vi "TEST.vi"() -> ()   [LabVIEW 2017]
uses:
  <vilib>/Utility/miscctls.llb/LVPointTypeDef.ctl
  <vilib>/Utility/miscctls.llb/LVBoundsTypeDef.ctl
  <vilib>/Utility/miscctls.llb/LVRectTypeDef.ctl
panel:
  in  "stop":bool
  out "PictureBox":picture
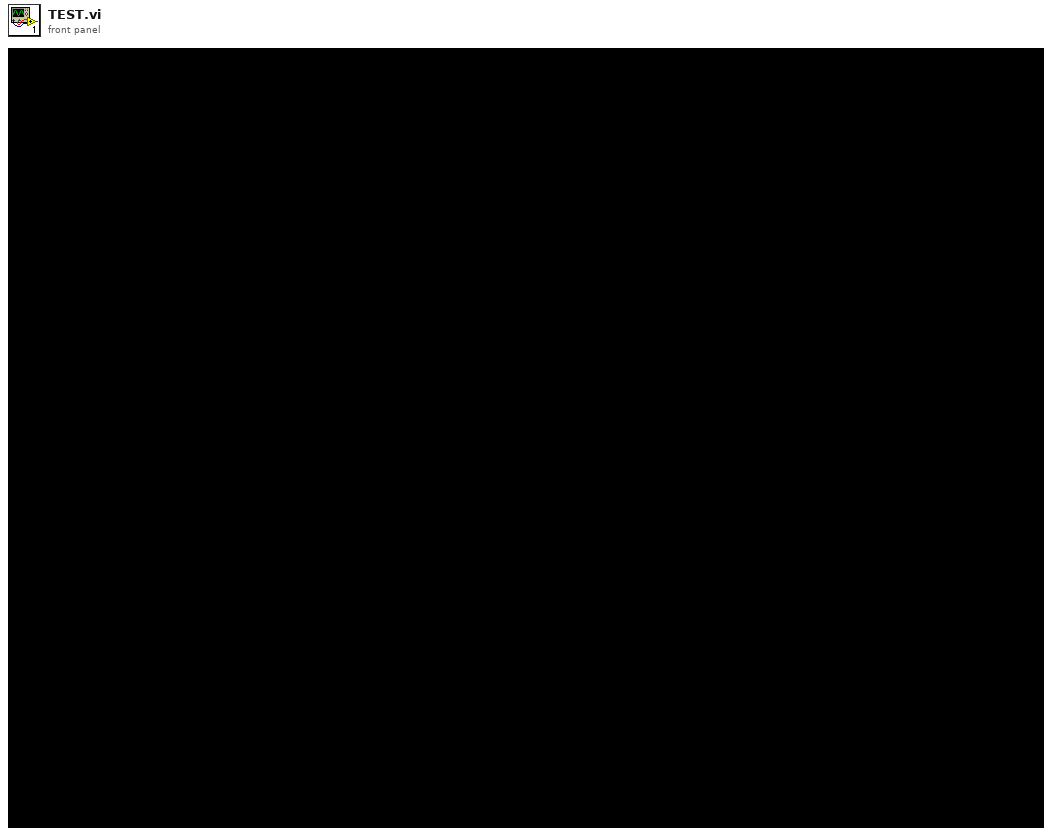
[diagram p1: front panel]
types:
  T1 = typedef "LVRectTypeDef.ctl" = cluster{"Left":i16, "Top":i16, "Right":i16, "Bottom":i16}
  T2 = typedef "LVBoundsTypeDef.ctl" = cluster{"Width":u32, "Height":u32}
  T3 = typedef "LVPointTypeDef.ctl" = cluster{"Horizontal":i16, "Vertical":i16}
  T4 = typedef "imagedata.ctl" = cluster{"image type":i32, "image depth":i32, "image":u8[], "mask":u8[], "colors":u32[], "Rectangle":cluster{"left":i16, "top":i16, "right":i16, "bottom":i16}}
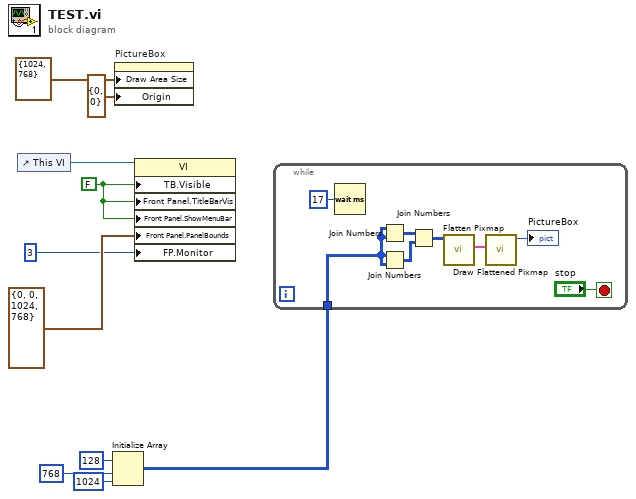
[diagram p0: block diagram]
diagram:
  w7 = FALSE ("Tool Bar:Visible")
  n1 = control-ref of="This VI"() -> (w8:refnum<vi>)
  n2 = Initialize Array(u8 128 ("element"), 768 ("dimension size"), 1024 ("dimension size")) -> (w1:u8[][])
  n3 = property on="PictureBox" class="Pict"("Draw Area Size"=T2 {"Width"=1024, "Height"=768}, "Origin"=T3 {"Horizontal"=0, "Vertical"=0}) -> ()  [unwired: 2 in, 2 out]
  n4 = property class="VI"(reference=w8, "TB.Visible"=w7, "Front Panel.TitleBarVis"=w7, "Front Panel.ShowMenuBar"=w7, "Front Panel.PanelBounds"=T1 {"Left"=0, "Top"=0, "Right"=1024, "Bottom"=768} ("Front Panel Window:Panel Bounds"), "FP.Monitor"=u16 3 ("Monitor")) -> ()  [unwired: 1 in, 2 out]
  n5 = while {
    tunnel: w1 -> [w11]
    stop <- "stop" stop-if-true
    n6 = Wait (ms)(milliseconds to wait=u32 17) -> ()  [unwired: 1 out]
    n7 = Join Numbers(hi=w11, lo=w11) -> ((hi.lo)=w14:u16[][])
    n8 = Join Numbers(hi=w11, lo=w11) -> ((hi.lo)=w13:u16[][])
    n9 = Join Numbers(hi=w14, lo=w13) -> ((hi.lo)=w12:u32[][])
    n10 = call <vilib>:"Flatten Pixmap.vi"("24-bit pixmap"=w12) -> ("image data"=w16:T4)  [unwired: 10 in]
    n11 = call <vilib>:"Draw Flattened Pixmap.vi"("image data"=w16) -> ("new picture"=→"PictureBox":picture)  [unwired: 8 in]
  }
